vi "Values of neighbours to bools.vi"(11 "Array in":u32[][](array[numeric])) -> (2 "Array":bool[][](array[boolean]), 3 "Array Waardes van de neighbours":u32[][](array[numeric]))   [LabVIEW 2013]
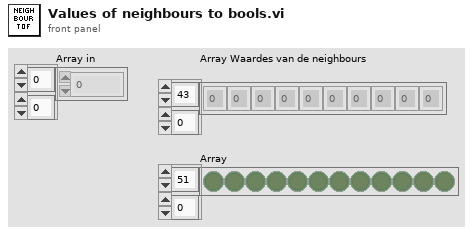
[diagram p1: front panel]
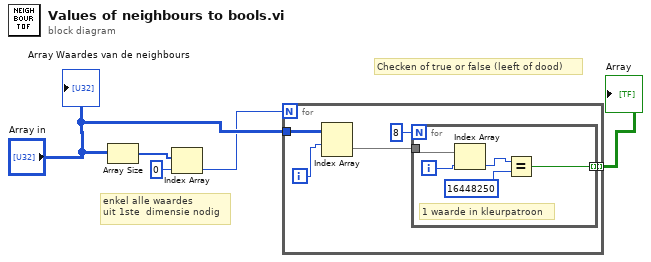
[diagram p0: block diagram]
diagram:
  # "enkel alle waardes\nuit 1ste  dimensie nodig"
  # "Checken of true or false (leeft of dood)"
  n1 = Array Size(array="Array in") -> (size(s)=w1:i32[])
  n2 = Index Array(array=w1, index=0) -> (element=w3:i32)
  n3 = for {
    N: w3 -> [_]
    tunnel: "Array in" -> [w10]
    tunnel: [w6] -> w5 mode=indexing
    i -> [w7]
    n4 = Index Array(array=w10, index (row)=w7) -> (element=w9:u32[])  [unwired: 1 in]
    n5 = for {
      N: 8 -> [_]
      tunnel: w9 -> [w15]
      tunnel: [w11] -> w6 mode=indexing
      i -> [w14]
      # "1 waarde in kleurpatroon"
      n6 = Index Array(array=w15, index=w14) -> (element=w13:u32)
      n7 = Equal?(x=w13, y=u32 16448250) -> (x = y?=w11:bool)
    }
  }
  "Array" <- w5
  "Array Waardes van de neighbours" <- "Array in"
